vi "Start Leak Check Cycle.vi"(8 "error in (no error)":errorcluster, 10 "Type of Cycle (0:Molbox1+)":i32(ring) items=["Molbox1+", "System"], 11 "VISA resource name":refnum<visa-resource-name>) -> (0 "error out":errorcluster, 3 "VISA resource name out":refnum<visa-resource-name>)   [LabVIEW 2023, in "Fluke Molbox 1 Plus.lvlib"]
doc: "Starts a molbox1+ or system leak check cycle. Both leak checks take 60 seconds to complete. At the end of the leak check, the molbox1+ is returned to its normal operating state.\n\nThe “ABORT” command can be used to stop a leak check cycle, clear out any\nprevious error messages, and return the molbox1+ to its normal operating state.\nWhile the leak check cycle is executing, a ‘b’ (“busy”) will appear in the 3rd\ncharacter position of the “FR” and the “SR” command replies."
uses:
  Fluke Molbox 1 Plus.lvlib
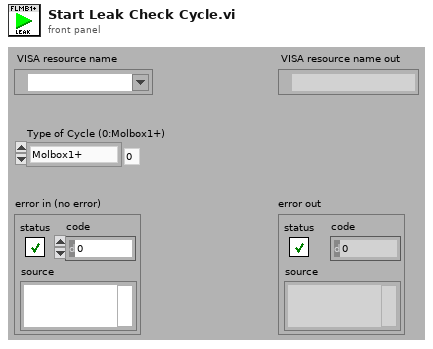
[diagram p1: front panel]
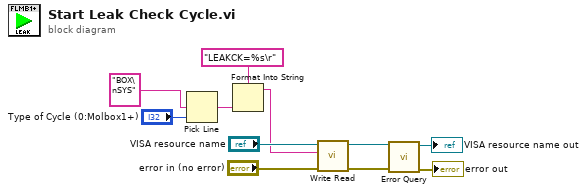
[diagram p0: block diagram]
diagram:
  n1 = Pick Line(multi-line string="BOX\nSYS", line index="Type of Cycle (0:Molbox1+)") -> (output string=w6:string)  [unwired: 1 in]
  n2 = Format Into String(format string="LEAKCK=%s\r", w6) -> (resulting string=w2:string)  [unwired: 2 in, 1 out]
  n3 = call "Write Read.vi"("error in (no error)"="error in (no error)", "Write String"=w2, "VISA resource name"="VISA resource name") -> ("error out"=w4:errorcluster, "VISA resource name out"=w5:refnum<visa-resource-name>)  [unwired: 6 in, 1 out]
  n4 = call "Error Query.vi"("error in (no error)"=w4, "VISA resource name"=w5) -> ("error out"=→"error out":errorcluster, "VISA resource name out"=→"VISA resource name out":refnum<visa-resource-name>)  [unwired: 6 in, 2 out]
